vi "Unzip.vi"   [LabVIEW 2020]
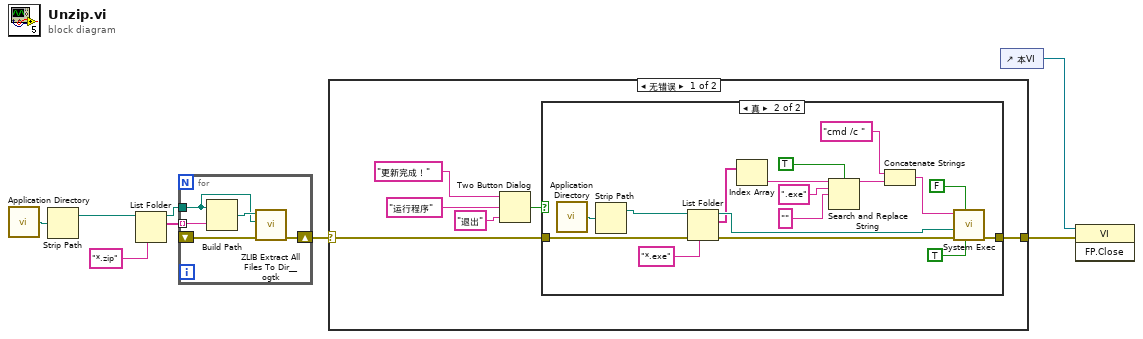
[diagram p0: block diagram]
diagram:
  n1 = call <vilib>:"Application Directory.vi"() -> ("Application Directory"=w4:path)
  n2 = Strip Path(path=w4) -> (stripped path=w3:path)  [unwired: 1 out]
  n3 = List Folder(path=w3, pattern="*.zip" ("类型")) -> (path out=w7:path, filenames=w6:string[])  [unwired: 2 in, 2 out]
  n4 = for {
    shift-right: [w12] -> w5
    shift-left: _ -> [w13]
    tunnel: w7 -> [w9]
    tunnel: w6 -> [w11] mode=indexing
    n5 = Build Path(base path=w9, name or relative path=w11) -> (appended path=w10:path)
    n6 = call <userlib>:"ZLIB Extract All Files To Dir__ogtk.vi"("error in (no error)"=w13, "root directory (archive name without ending)"=w9, "archive name (file dialog)"=w10) -> ("error out"=w12:errorcluster)  [unwired: 6 in, 2 out]
  }
  n7 = case shown="无错误" w5 {
    selector: w5 -> [w19 w38]
    tunnel: [w18 w38] -> w1
    frame No Error {
      n8 = Two Button Dialog(message="更新完成！" ("消息"), 1:"退出" ("F按钮名称（“取消”）"), 2:"运行程序" ("T按钮名称（“确定”）")) -> (T button?=w16:bool)
      n9 = case shown="真" w16 {
        tunnel: w19 -> [w20 w36]
        tunnel: [w20 w27] -> w18
        frame False {
        }
        frame True {
          n10 = call <vilib>:"Application Directory.vi"() -> ("Application Directory"=w33:path)
          n11 = Strip Path(path=w33) -> (stripped path=w32:path)  [unwired: 1 out]
          n12 = List Folder(path=w32, pattern="*.exe" ("类型"), error in=w36) -> (path out=w35:path, filenames=w34:string[], error out=w28:errorcluster)  [unwired: 1 in, 1 out]
          n13 = Index Array(array=w34) -> (element=w26:string)  [unwired: 1 in]
          n14 = Search and Replace String(case sensitive?=TRUE ("忽略大小写？(F)"), input string=w26, search string=".exe" ("搜索字符串"), replace string="" ("替换字符串(\"\")")) -> (result string=w22:string)  [unwired: 4 in, 3 out]
          n15 = Concatenate Strings("cmd /c " ("字符串"), w22) -> (w30:string)
          n16 = call <vilib>:"System Exec.vi"("run minimized? (F)"=TRUE, "wait until completion? (T)"=FALSE, "error in (no error)"=w28, "working directory"=w35, "command line"=w30) -> ("error out"=w27:errorcluster)  [unwired: 3 in, 3 out]
        }
      }
    }
    frame Error {
    }
  }
  n17 = control-ref of="本VI"() -> (w2:refnum<vi>)
  n18 = invoke class="VI" method="FP.Close"(reference=w2, error in=w1) -> ()  [unwired: 1 in, 3 out]
